vi "Orifice_Z.vi"(8 "Model":T3=enum."Gallas", 9 "Thermo and Transport Properties":T1, 10 "SJ Geometry":T2, 11 "Omega":dbl=1500000.0) -> (0 "Ku":dbl=137.85709652529974, 1 "Km":dbl=0.7513638139341703, 2 "Kr":dbl=137.85709652529974, 3 "Zo":cdb=1678525.5334913884+922226140.0501939i)   [LabVIEW 2012]
uses:
  Model.ctl
  Utilities/fluid_properties/fluid_properties.ctl
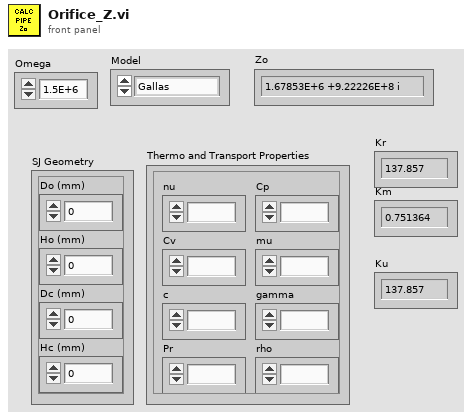
[diagram p1: front panel]
types:
  T1 = typedef "fluid_properties.ctl" = cluster{"nu":dbl, "c":dbl, "Pr":dbl, "Cp":dbl, "Cv":dbl, "gamma":dbl, "mu":dbl, "rho":dbl}
  T2 = cluster{"Do (mm)":dbl, "Ho (mm)":dbl, "Dc (mm)":dbl, "Hc (mm)":dbl}
  T3 = typedef "Model.ctl" = enum16{"Martin", "Tang", "Gallas", "Persoon"}
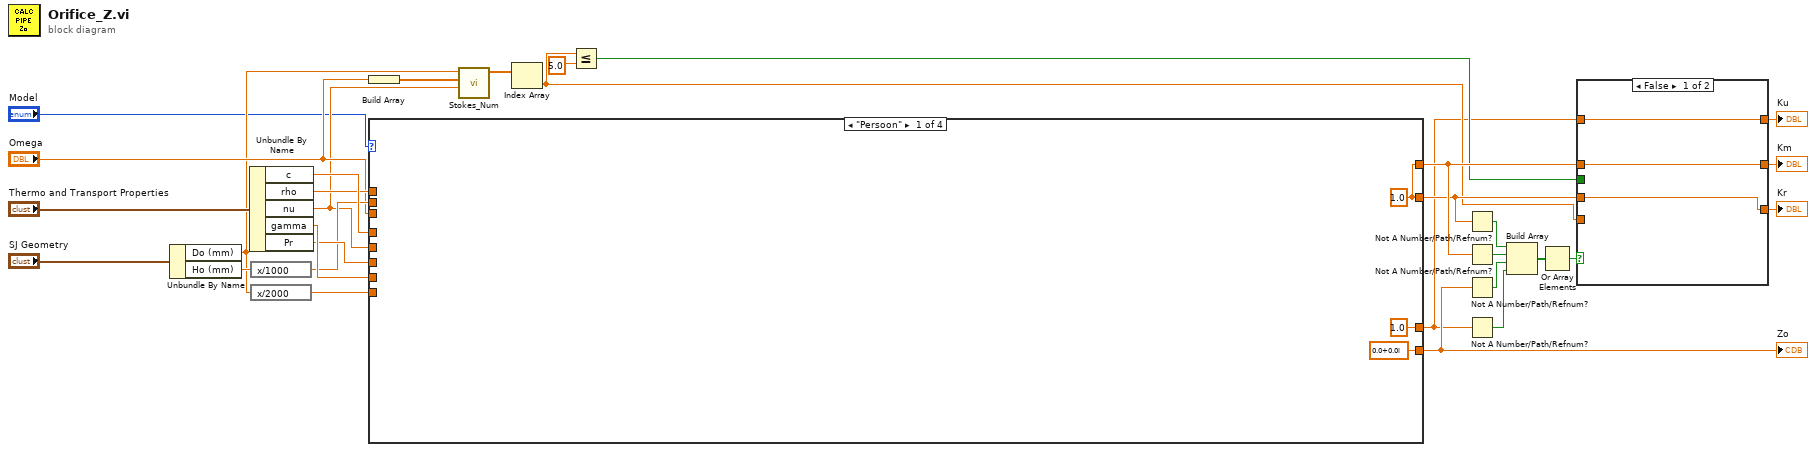
[diagram p0: block diagram]
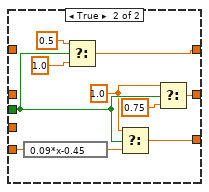
[diagram p2: hidden frame]
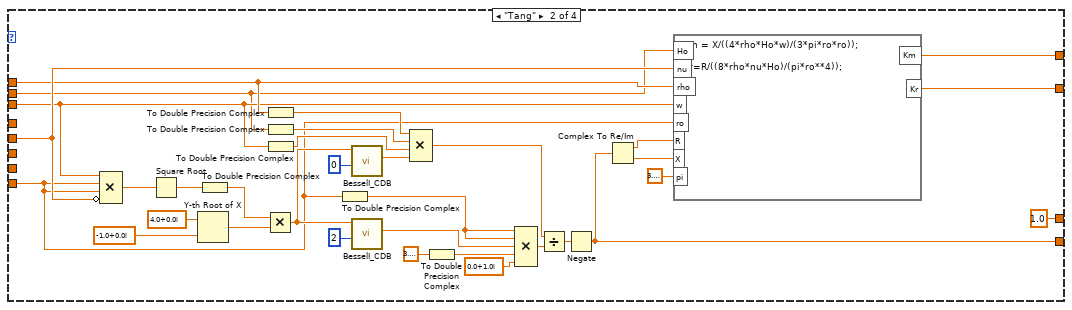
[diagram p3: hidden frame]
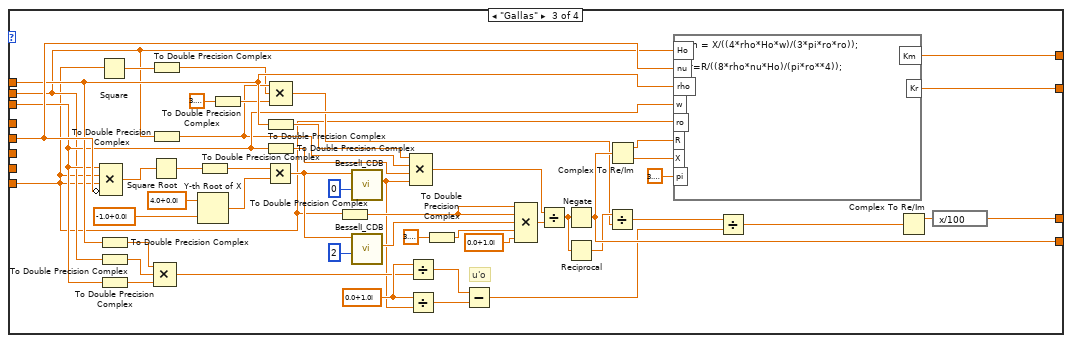
[diagram p4: hidden frame]
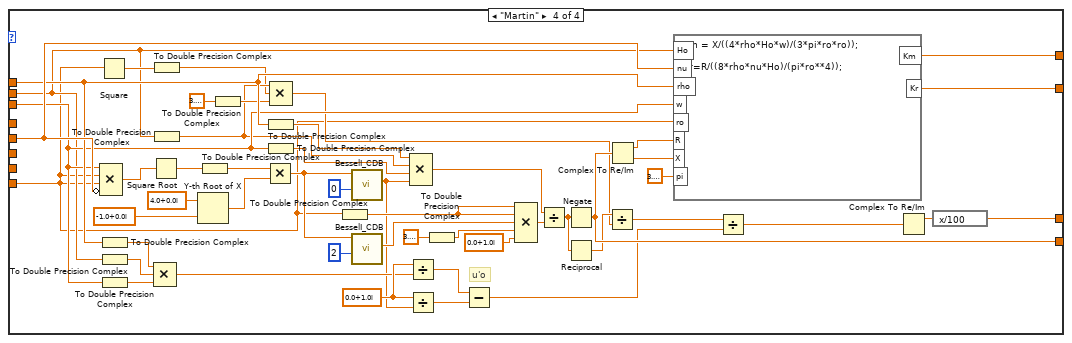
[diagram p5: hidden frame]
diagram:
  n1 = Unbundle By Name("SJ Geometry") -> ("Do (mm)"=w10:dbl, "Ho (mm)"=w29:dbl)
  n2 = Unbundle By Name("Thermo and Transport Properties") -> ("c"=w26:dbl, "rho"=w25:dbl, "nu"=w9:dbl, "gamma"=w28:dbl, "Pr"=w27:dbl)
  n3 = expression code="x/1000"(w29) -> (w23:dbl)
  n4 = expression code="x/2000"(w10) -> (w24:dbl)
  n5 = Build Array("Omega") -> (w11:dbl[])
  n6 = case shown="\"Persoon\"" "Model" {
    tunnel: [cdb 0.0+0.0i w50 w100 w150] -> w5
    tunnel: w9 -> [_ w49 w99 w149]
    tunnel: w25 -> [_ w43 w82 w132]
    tunnel: w23 -> [_ w39 w72 w122]
    tunnel: "Omega" -> [_ w42 w81 w131]
    tunnel: w24 -> [_ w36 w68 w118]
    tunnel: [w33 w47 w97 w147] -> w13
    tunnel: [w33 w46 w96 w146] -> w15
    tunnel: w28 -> [_ _ _ _]
    tunnel: w27 -> [_ _ _ _]
    tunnel: w26 -> [_ _ _ _]
    tunnel: [1.0 1.0 w83 w133] -> w2
    frame "Persoon" {
      w33 = 1.0 ("Km")
    }
    frame "Tang" {
      n7 = Compound Arithmetic op=MULTIPLY(w42, w36, w36, invert w49) -> (w66:dbl)
      n8 = Square Root(x=w66) -> (sqrt(x)=w67:dbl)
      n9 = Y-th Root of X(1:cdb -1.0+0.0i ("x"), 2:cdb 4.0+0.0i ("y")) -> (0:w63:cdb)
      n10 = To Double Precision Complex(1:w67) -> (0:w62:cdb)
      n11 = Multiply(x=w62, y=w63) -> (x*y=w59:cdb)
      n12 = To Double Precision Complex(1:w43) -> (0:w58:cdb)
      n13 = To Double Precision Complex(1:w39) -> (0:w40:cdb)
      n14 = To Double Precision Complex(1:w42) -> (0:w57:cdb)
      n15 = To Double Precision Complex(1:w36) -> (0:w52:cdb)
      n16 = call "BesselI_CDB.vi"("n"=0, "z"=w59) -> ("BesselIn(z)"=w37:cdb)  [unwired: 9 in]
      n17 = call "BesselI_CDB.vi"("n"=2, "z"=w59) -> ("BesselIn(z)"=w53:cdb)  [unwired: 9 in]
      n18 = Compound Arithmetic op=MULTIPLY(w58, w40, w57, w37) -> (w38:cdb)
      n19 = To Double Precision Complex(1:3.141592653589793) -> (0:w54:cdb)
      n20 = Compound Arithmetic op=MULTIPLY(w52, w52, w53, w54, cdb 0.0+1.0i ("x")) -> (w51:cdb)
      n21 = Divide(x=w38, y=w51) -> (x/y=w41:cdb)
      n22 = Negate(x=w41) -> (-x=w50:cdb)
      n23 = Complex To Re/Im(x + iy=w50) -> (x=w44:dbl, y=w48:dbl)
      n24 = formula code="Km = X/((4*rho*Ho*w)/(3*pi*ro*ro));\n\nKr=R/((8*rho*nu*Ho)/(pi*ro**4));"("nu"=w49, "rho"=w43, "Ho"=w39, "w"=w42, "ro"=w36, "R"=w44, "X"=w48, "pi"=3.141592653589793) -> ("Km"=w46:dbl, "Kr"=w47:dbl)
    }
    frame "Gallas" {
      w88 = cdb 0.0+1.0i ("x")
      # "u'o"
      n25 = Square(x=w68) -> (x^2=w74:dbl)
      n26 = Compound Arithmetic op=MULTIPLY(w81, w68, w68, invert w99) -> (w116:dbl)
      n27 = To Double Precision Complex(1:w82) -> (0:w91:cdb)
      n28 = To Double Precision Complex(1:w72) -> (0:w92:cdb)
      n29 = To Double Precision Complex(1:w81) -> (0:w93:cdb)
      n30 = Square Root(x=w116) -> (sqrt(x)=w117:dbl)
      n31 = To Double Precision Complex(1:w74) -> (0:w73:cdb)
      n32 = To Double Precision Complex(1:w72) -> (0:w75:cdb)
      n33 = Compound Arithmetic op=MULTIPLY(w91, w92, w93) -> (w87:cdb)
      n34 = Y-th Root of X(1:cdb -1.0+0.0i ("x"), 2:cdb 4.0+0.0i ("y")) -> (0:w113:cdb)
      n35 = To Double Precision Complex(1:w117) -> (0:w112:cdb)
      n36 = To Double Precision Complex(1:3.141592653589793) -> (0:w78:cdb)
      n37 = Multiply(x=w112, y=w113) -> (x*y=w109:cdb)
      n38 = To Double Precision Complex(1:w82) -> (0:w108:cdb)
      n39 = To Double Precision Complex(1:w81) -> (0:w107:cdb)
      n40 = Compound Arithmetic op=MULTIPLY(w75, w73, w78) -> (w76:cdb)
      n41 = To Double Precision Complex(1:w68) -> (0:w102:cdb)
      n42 = call "BesselI_CDB.vi"("n"=0, "z"=w109) -> ("BesselIn(z)"=w69:cdb)  [unwired: 9 in]
      n43 = call "BesselI_CDB.vi"("n"=2, "z"=w109) -> ("BesselIn(z)"=w103:cdb)  [unwired: 9 in]
      n44 = Divide(x=w88, y=w87) -> (x/y=w89:cdb)
      n45 = Divide(x=w88, y=w69) -> (x/y=w90:cdb)
      n46 = Compound Arithmetic op=MULTIPLY(w108, w75, w107, w69) -> (w70:cdb)
      n47 = To Double Precision Complex(1:3.141592653589793) -> (0:w104:cdb)
      n48 = Subtract(x=w89, y=w90) -> (x-y=w85:cdb)
      n49 = Compound Arithmetic op=MULTIPLY(w102, w102, w103, w104, cdb 0.0+1.0i ("x")) -> (w101:cdb)
      n50 = Divide(x=w70, y=w101) -> (x/y=w80:cdb)
      n51 = Negate(x=w80) -> (-x=w100:cdb)
      n52 = Reciprocal(x=w80) -> (1/x=w79:cdb)
      n53 = Divide(x=w79, y=w76) -> (x/y=w71:cdb)
      n54 = Complex To Re/Im(x + iy=w100) -> (x=w94:dbl, y=w98:dbl)
      n55 = formula code="Km = X/((4*rho*Ho*w)/(3*pi*ro*ro));\n\nKr=R/((8*rho*nu*Ho)/(pi*ro**4));"("nu"=w99, "rho"=w82, "Ho"=w72, "w"=w81, "ro"=w68, "R"=w94, "X"=w98, "pi"=3.141592653589793) -> ("Km"=w96:dbl, "Kr"=w97:dbl)
      n56 = Divide(x=w71, y=w85) -> (x/y=w84:cdb)
      n57 = Complex To Re/Im(x + iy=w84) -> (x=w86:dbl)  [unwired: 1 out]
      n58 = expression code="x/100"(w86) -> (w83:dbl)
    }
    frame "Martin" {
      w138 = cdb 0.0+1.0i ("x")
      # "u'o"
      n59 = Square(x=w118) -> (x^2=w124:dbl)
      n60 = Compound Arithmetic op=MULTIPLY(w131, w118, w118, invert w149) -> (w166:dbl)
      n61 = To Double Precision Complex(1:w132) -> (0:w141:cdb)
      n62 = To Double Precision Complex(1:w122) -> (0:w142:cdb)
      n63 = To Double Precision Complex(1:w131) -> (0:w143:cdb)
      n64 = Square Root(x=w166) -> (sqrt(x)=w167:dbl)
      n65 = To Double Precision Complex(1:w124) -> (0:w123:cdb)
      n66 = To Double Precision Complex(1:w122) -> (0:w125:cdb)
      n67 = Compound Arithmetic op=MULTIPLY(w141, w142, w143) -> (w137:cdb)
      n68 = Y-th Root of X(1:cdb -1.0+0.0i ("x"), 2:cdb 4.0+0.0i ("y")) -> (0:w163:cdb)
      n69 = To Double Precision Complex(1:w167) -> (0:w162:cdb)
      n70 = To Double Precision Complex(1:3.141592653589793) -> (0:w128:cdb)
      n71 = Multiply(x=w162, y=w163) -> (x*y=w159:cdb)
      n72 = To Double Precision Complex(1:w132) -> (0:w158:cdb)
      n73 = To Double Precision Complex(1:w131) -> (0:w157:cdb)
      n74 = Compound Arithmetic op=MULTIPLY(w125, w123, w128) -> (w126:cdb)
      n75 = To Double Precision Complex(1:w118) -> (0:w152:cdb)
      n76 = call "BesselI_CDB.vi"("n"=0, "z"=w159) -> ("BesselIn(z)"=w119:cdb)  [unwired: 9 in]
      n77 = call "BesselI_CDB.vi"("n"=2, "z"=w159) -> ("BesselIn(z)"=w153:cdb)  [unwired: 9 in]
      n78 = Divide(x=w138, y=w137) -> (x/y=w139:cdb)
      n79 = Divide(x=w138, y=w119) -> (x/y=w140:cdb)
      n80 = Compound Arithmetic op=MULTIPLY(w158, w125, w157, w119) -> (w120:cdb)
      n81 = To Double Precision Complex(1:3.141592653589793) -> (0:w154:cdb)
      n82 = Subtract(x=w139, y=w140) -> (x-y=w135:cdb)
      n83 = Compound Arithmetic op=MULTIPLY(w152, w152, w153, w154, cdb 0.0+1.0i ("x")) -> (w151:cdb)
      n84 = Divide(x=w120, y=w151) -> (x/y=w130:cdb)
      n85 = Negate(x=w130) -> (-x=w150:cdb)
      n86 = Reciprocal(x=w130) -> (1/x=w129:cdb)
      n87 = Divide(x=w129, y=w126) -> (x/y=w121:cdb)
      n88 = Complex To Re/Im(x + iy=w150) -> (x=w144:dbl, y=w148:dbl)
      n89 = formula code="Km = X/((4*rho*Ho*w)/(3*pi*ro*ro));\n\nKr=R/((8*rho*nu*Ho)/(pi*ro**4));"("nu"=w149, "rho"=w132, "Ho"=w122, "w"=w131, "ro"=w118, "R"=w144, "X"=w148, "pi"=3.141592653589793) -> ("Km"=w146:dbl, "Kr"=w147:dbl)
      n90 = Divide(x=w121, y=w135) -> (x/y=w134:cdb)
      n91 = Complex To Re/Im(x + iy=w134) -> (x=w136:dbl)  [unwired: 1 out]
      n92 = expression code="x/100"(w136) -> (w133:dbl)
    }
  }
  "Zo" <- w5
  n93 = call "Stokes_Num.vi"("nu"=w9, "omega"=w11, "Do (mm)"=w10) -> ("Stokes number"=w8:dbl[])  [unwired: 8 in]
  n94 = Index Array(array=w8) -> (element=w4:dbl)  [unwired: 1 in]
  n95 = Less Or Equal?(x=w4, y=5.0) -> (x <= y?=w6:bool)
  n96 = Not A Number/Path/Refnum?(number/path/refnum=w13) -> (NaN/Path/Refnum?=w19:bool)
  n97 = Not A Number/Path/Refnum?(number/path/refnum=w15) -> (NaN/Path/Refnum?=w20:bool)
  n98 = Not A Number/Path/Refnum?(number/path/refnum=w5) -> (NaN/Path/Refnum?=w21:bool)
  n99 = Not A Number/Path/Refnum?(number/path/refnum=w2) -> (NaN/Path/Refnum?=w22:bool)
  n100 = Build Array(w19, w20, w21, w22) -> (w18:bool[])
  n101 = Or Array Elements(Boolean array=w18) -> (logical OR=w17:bool)
  n102 = case shown="False" w17 {
    tunnel: [w170 w180] -> w16
    tunnel: w15 -> [w170 _]
    tunnel: [w169 w178] -> w14
    tunnel: w13 -> [w169 _]
    tunnel: [w168 w179] -> w3
    tunnel: w2 -> [w168 _]
    tunnel: w6 -> [_ w177]
    tunnel: w4 -> [_ w172]
    frame False {
    }
    frame True {
      w174 = 1.0 ("t")
      n103 = expression code="0.09*x-0.45"(w172) -> (w171:dbl)
      n104 = Select(t=0.5, s=w177, f=1.0 ("t")) -> (s? t:f=w179:dbl)
      n105 = Select(t=w174, s=w177, f=w171) -> (s? t:f=w178:dbl)
      n106 = Select(t=w174, s=w177, f=0.75) -> (s? t:f=w180:dbl)
    }
  }
  "Kr" <- w14
  "Km" <- w16
  "Ku" <- w3
